vi "Re-Populate Tree for Filter.vi"(6 "Indent level":i32, 8 "error in":errorcluster, 9 "Data in":string[](array[string]), 10 "Tags map":refnum<vi>, 11 "TreeControl in":refnum<vi>) -> (0 "error out":errorcluster)   [LabVIEW 2025, in "CAN-LIN Raw Bus Capture UI.lvlib"]
uses:
  CAN-LIN Raw Bus Capture UI.lvlib
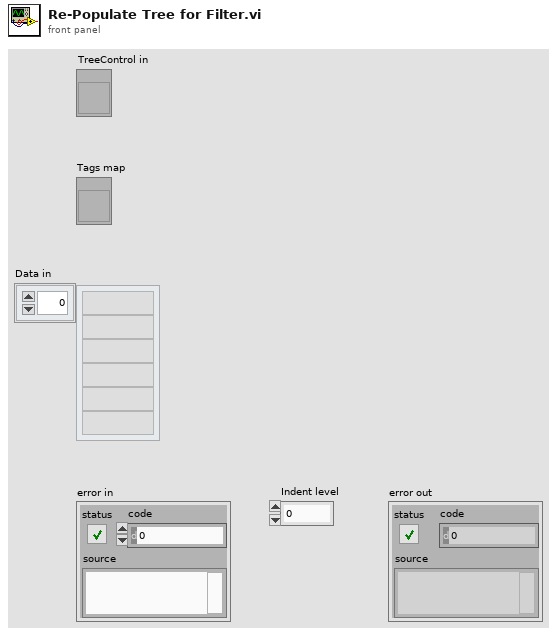
[diagram p1: front panel]
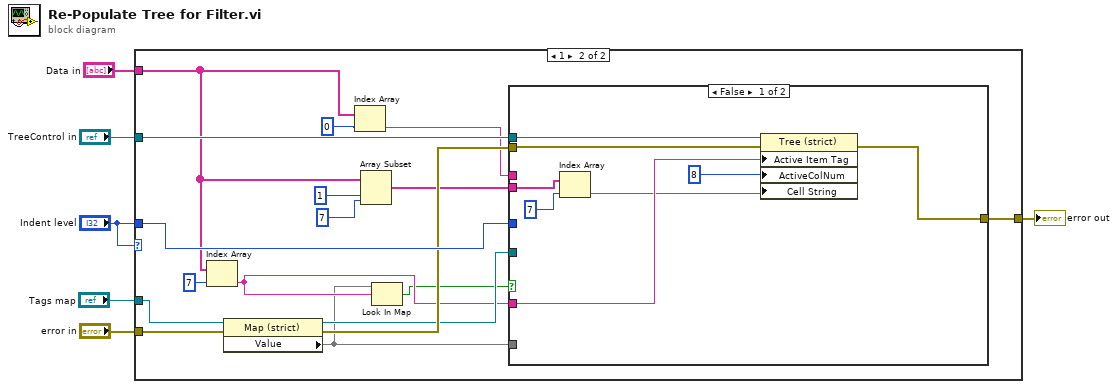
[diagram p0: block diagram]
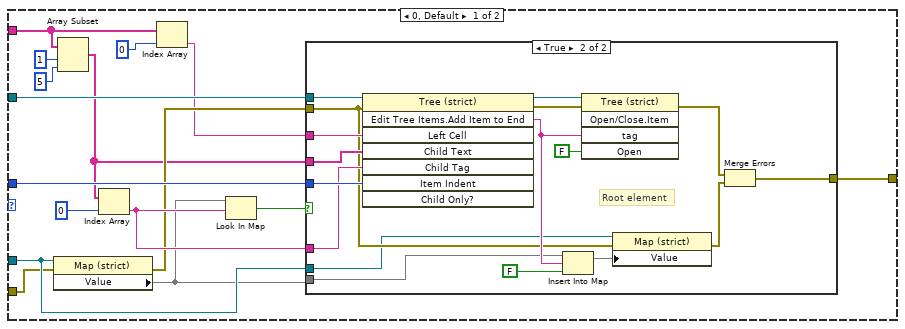
[diagram p2: hidden frame]
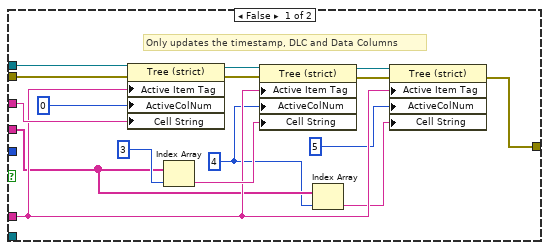
[diagram p3: hidden frame]
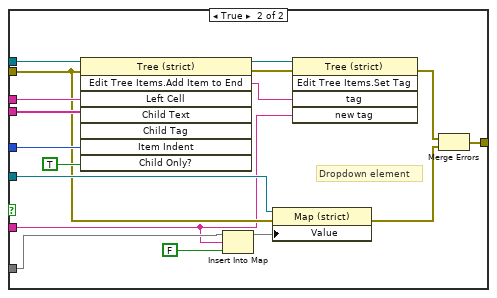
[diagram p4: hidden frame]
diagram:
  n1 = case shown="1" "Indent level" {
    tunnel: "Indent level" -> [w22 w72]
    tunnel: [w21 w71] -> w6
    tunnel: "TreeControl in" -> [w17 w69]
    tunnel: "error in" -> [w16 w67]
    tunnel: "Tags map" -> [w19 w68]
    tunnel: "Data in" -> [w9 w58]
    frame 0, Default {
      n2 = property class="Map (strict)"(reference=w19, error in=w16) -> (error out=w15:errorcluster, "Value"=w13:map{string, bool})  [unwired: 1 out]
      n3 = Array Subset(array=w9, index=1, length=5) -> (w8:string[])
      n4 = Index Array(array=w8, index=0) -> (element=w18:string)
      n5 = Index Array(array=w9, index=0) -> (element=w7:string)
      n6 = Look In Map(map=w13, key=w18) -> (key not found?=w14:bool)  [unwired: 1 in, 1 out]
      n7 = case shown="True" w14 {
        tunnel: w17 -> [w38 w52]
        tunnel: w15 -> [w37 w41]
        tunnel: w22 -> [_ w51]
        tunnel: [w25 w42] -> w21
        tunnel: w7 -> [w35 w50]
        tunnel: w8 -> [w27 w49]
        tunnel: w18 -> [w28 w48]
        tunnel: w19 -> [_ w40]
        tunnel: w13 -> [_ w39]
        frame False {
          w24 = 4 ("index")
          # "Only updates the timestamp, DLC and Data Columns"
          n8 = property class="Tree (strict)"(reference=w38, error in=w37, "Active Item Tag"=w28, "ActiveColNum"=0 ("Active Cell:Active Column Number"), "Cell String"=w35) -> (reference out=w34:refnum<vi>, error out=w33:errorcluster)
          n9 = Index Array(array=w27, index=3 ("Active Cell:Active Column Number")) -> (element=w31:string)
          n10 = property class="Tree (strict)"(reference=w34, error in=w33, "Active Item Tag"=w28, "ActiveColNum"=w24, "Cell String"=w31) -> (reference out=w30:refnum<vi>, error out=w29:errorcluster)
          n11 = Index Array(array=w27, index=w24) -> (element=w26:string)
          n12 = property class="Tree (strict)"(reference=w30, error in=w29, "Active Item Tag"=w28, "ActiveColNum"=5 ("Active Cell:Active Column Number"), "Cell String"=w26) -> (error out=w25:errorcluster)  [unwired: 1 out]
        }
        frame True {
          # "Root element"
          n13 = invoke on="Invoke Node" class="Tree (strict)" method="Edit Tree Items.Add Item to End"(reference=w52, error in=w41, "Left Cell"=w50, "Child Text"=w49, "Child Tag"=w48, "Item Indent"=w51) -> (reference out=w53:refnum<vi>, error out=w55:errorcluster, "Edit Tree Items:Add Item to End"=w47:string)  [unwired: 2 in, 5 out]
          n14 = Insert Into Map(map in=w39, key=w47, value=FALSE) -> (map out=w45:map{string, bool})  [unwired: 2 out]
          n15 = invoke on="Invoke Node" class="Tree (strict)" method="Open/Close.Item"(reference=w53, error in=w55, "tag"=w47, "Open"=FALSE ("Open?")) -> (error out=w44:errorcluster)  [unwired: 1 in, 4 out]
          n16 = property class="Map (strict)"(reference=w40, error in=w41, "Value"=w45) -> (error out=w43:errorcluster)  [unwired: 1 out]
          n17 = Merge Errors(w44, w43) -> (w42:errorcluster)
        }
      }
    }
    frame 1 {
      n18 = Index Array(array=w58, index=7) -> (element=w64:string)
      n19 = property class="Map (strict)"(reference=w68, error in=w67) -> (reference out=w65:refnum<vi>, error out=w66:errorcluster, "Value"=w63:map{string, bool})
      n20 = Index Array(array=w58, index=0) -> (element=w60:string)
      n21 = Array Subset(array=w58, index=1, length=7) -> (w59:string[])
      n22 = Look In Map(map=w63, key=w64) -> (key not found?=w62:bool)  [unwired: 1 in, 1 out]
      n23 = case shown="False" w62 {
        tunnel: w72 -> [_ w97]
        tunnel: [w80 w82] -> w71
        tunnel: w60 -> [_ w96]
        tunnel: w59 -> [w75 w92]
        tunnel: w69 -> [w78 w91]
        tunnel: w64 -> [w79 w81]
        tunnel: w66 -> [w77 w85]
        tunnel: w63 -> [_ w87]
        tunnel: w65 -> [_ w86]
        frame False {
          n24 = Index Array(array=w75, index=7) -> (element=w73:string)
          n25 = property class="Tree (strict)"(reference=w78, error in=w77, "Active Item Tag"=w79, "ActiveColNum"=8 ("Active Cell:Active Column Number"), "Cell String"=w73) -> (error out=w80:errorcluster)  [unwired: 1 out]
        }
        frame True {
          # "Dropdown element"
          n26 = invoke on="Invoke Node" class="Tree (strict)" method="Edit Tree Items.Add Item to End"(reference=w91, error in=w85, "Left Cell"=w96, "Child Text"=w92, "Item Indent"=w97, "Child Only?"=TRUE) -> (reference out=w93:refnum<vi>, error out=w94:errorcluster, "Edit Tree Items:Add Item to End"=w95:string)  [unwired: 2 in, 5 out]
          n27 = Insert Into Map(map in=w87, key=w81, value=FALSE) -> (map out=w88:map{string, bool})  [unwired: 2 out]
          n28 = property class="Map (strict)"(reference=w86, error in=w85, "Value"=w88) -> (error out=w84:errorcluster)  [unwired: 1 out]
          n29 = invoke on="Invoke Node" class="Tree (strict)" method="Edit Tree Items.Set Tag"(reference=w93, error in=w94, "tag"=w95, "new tag"=w81) -> (error out=w83:errorcluster)  [unwired: 1 in, 4 out]
          n30 = Merge Errors(w83, w84) -> (w82:errorcluster)
        }
      }
    }
  }
  "error out" <- w6
